vi "MSE.vi"(2 "X Values":dbl[](array[numeric]) format="%0.2f", 3 "Y Values":dbl[](array[numeric]) format="%0.2f") -> (0 "error":i32, 1 "mse":dbl format="%0.2f")   [LabVIEW 2024, in "NI_AALPro.lvlib"]
doc: "<p>Computes the mean square error (<strong>mse</strong>) of the input sequences <strong>X Values</strong> and <strong>Y Values</strong>.</p>"
uses:
  NI_AALPro.lvlib
  <resource>/lvanlys.dll
panel:
  # "Mean Square Error"
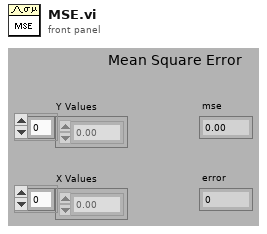
[diagram p1: front panel]
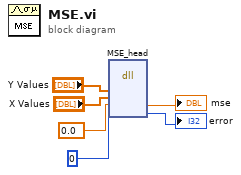
[diagram p0: block diagram]
diagram:
  n1 = dll-call lib="C:/Program Files (x86)/National Instruments/LabVIEW 2024/resource/lvanlys.*" fn="MSE_head"("Y Values"="Y Values", "X Values"="X Values", "output param"=0.0, "output param"=0) -> ("output param"=→"mse":dbl, "output param"=→"error":i32)  [unwired: 6 in, 2 out]
